vi "MultiScanDrift.vi"() -> ()   [LabVIEW 2014]
uses:
  <userlib>/Nanonis Prog Interface V5/Nanonis Prog Interface.lvlib
  shared/CorrelImages (SubVI)Single.vi
panel:
  in  "DC On":bool
  out "Y drift":i32
  out "X drift":i32
  in  "PLL switch delay":dbl=0.5 format="%_3p"
  out "DC active":bool
  in  "Drift correction Pixels":i32=256
  in  "Img Current":sgl=2.5e-11 format="%#_6p"
  in  "Img Bias (V)":sgl=0.02 format="%_2p"
  in  "Forward Speed":sgl=5e-10 format="%#_6p"
  in  "Backward Speed":sgl=8e-08 format="%#_6p"
  in  "Img Speed":sgl=3e-08 format="%#_6p"
  in  "Channel index (0-23)":u8(ring) items=["Current"=0, "Z (m)"=14]
  in  "Settling time (s)":dbl=0.7 format="%#_6p"
  in  "img bias":bool=TRUE
  in  "img bias":dbl=-0.0012 format="%#_6p"
  in  "img delay (s)":u32=1
  out "tipLift":dbl=1e-10 format="%#_6p"
  in  "TipLiftList":i32(listbox)
  in  "Const Height":bool=TRUE
  in  "CurrentList":i32(listbox)
  in  "BiasList":i32(listbox)
  out "Current":dbl=2.5e-11 format="%#_6p"
  out "Bias":dbl=0.02 format="%#_6p"
  # "Turn continuous scan off"
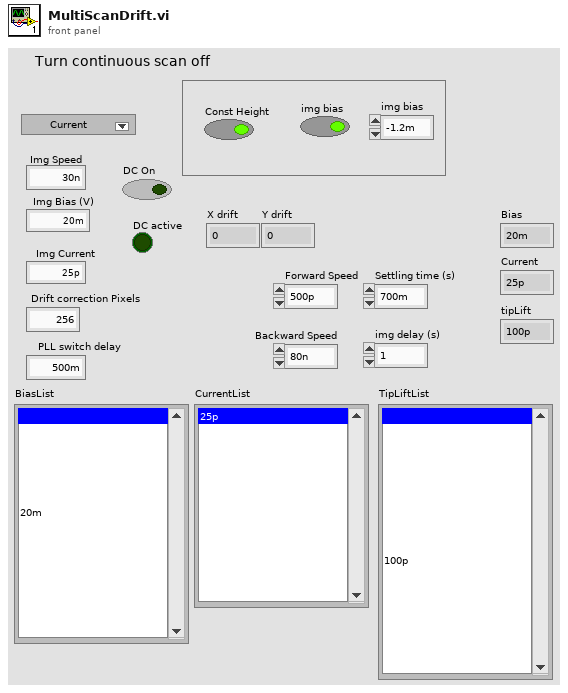
[diagram p1: front panel]
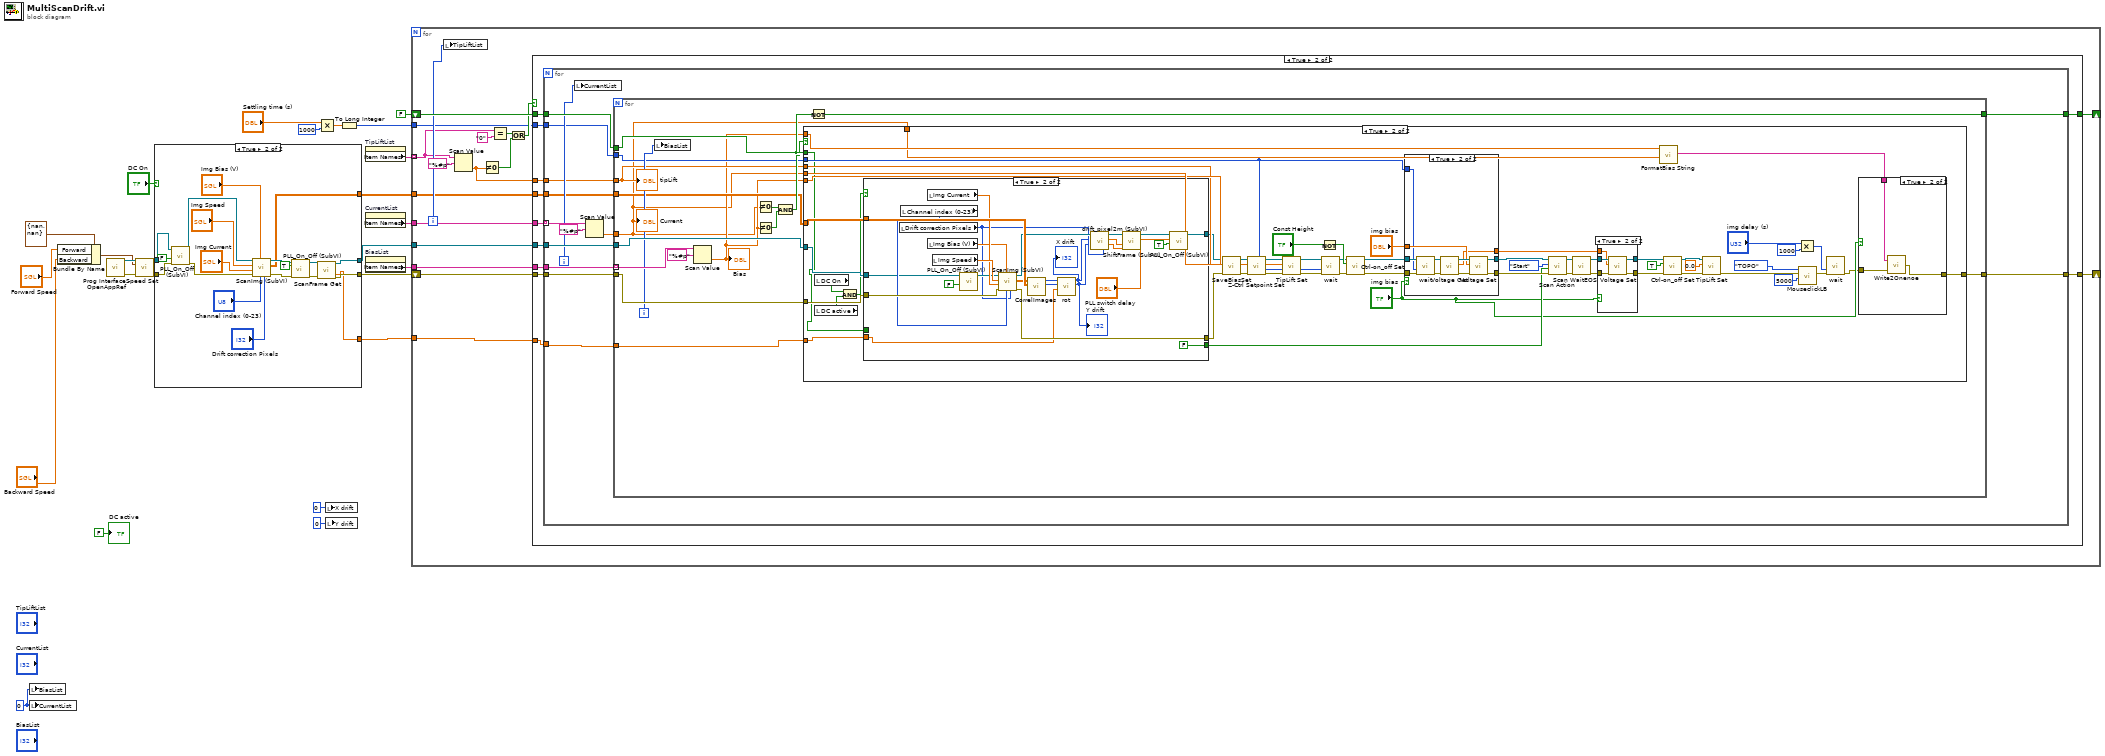
[diagram p0: block diagram]
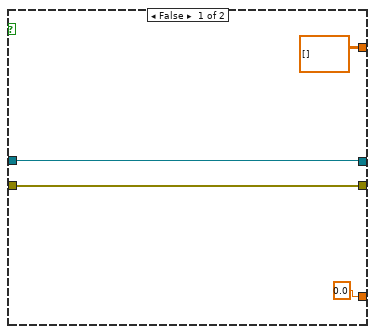
[diagram p2: hidden frame]
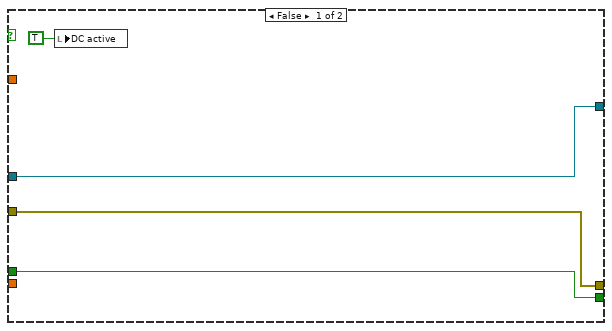
[diagram p6: hidden frame]
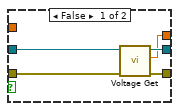
[diagram p8: hidden frame]
diagram:
  w25 = 0 ("BiasList")
  n1 = local write "BiasList"(w25) -> ()
  n2 = local write "CurrentList"(w25) -> ()
  n3 = Bundle By Name(cluster=cluster{"Forward":sgl, "Backward":sgl} {"Forward"=nan, "Backward"=nan} ("Speed (m/s)"), "Forward"="Forward Speed", "Backward"="Backward Speed") -> (w9:cluster{"Forward":sgl, "Backward":sgl})
  n4 = call <userlib>:"Prog Interface - OpenAppRef.vi"() -> ("Error out"=w10:errorcluster, "Application reference"=w11:refnum<vi>)  [unwired: 6 in]
  n5 = call <userlib>:"Speed Set.vi"("Application ref in"=w11, "Speed (m/s)"=w9, "error in (no error)"=w10) -> ("Application ref out"=w7:refnum<vi>, "error out"=w6:errorcluster)  [unwired: 11 in]
  n6 = case shown="True" "DC On" {
    tunnel: [w28 w32] -> w13
    tunnel: [w27 w31] -> w12
    tunnel: [dbl[][] [] ("Img") w41] -> w8
    tunnel: w7 -> [w28 w40]
    tunnel: w6 -> [w27 w38]
    tunnel: [sgl 0.0 ("Angle (deg)") w30] -> w1
    frame False {
    }
    frame True {
      n7 = call "PLL_On_Off (SubVI).vi"("error in (no error)"=w38, "Output ON/OFF (F=OFF)"=FALSE, "Application in"=w40) -> ("error out"=w37:errorcluster, "Application out"=w39:refnum<vi>)  [unwired: 7 in]
      n8 = call "ScanImg (SubVI).vi"("pixel"="Drift correction Pixels", "Channel index (0-23)"="Channel index (0-23)", "Bias (V)"="Img Bias (V)", "error in (no error)"=w37, "Current"="Img Current", "Img Speed"="Img Speed", "Application in"=w39) -> ("error out"=w44:errorcluster, "Img"=w41:dbl[][], "Application out"=w45:refnum<vi>)  [unwired: 2 in]
      n9 = call "PLL_On_Off (SubVI).vi"("error in (no error)"=w44, "Output ON/OFF (F=OFF)"=TRUE, "Application in"=w45) -> ("error out"=w33:errorcluster, "Application out"=w34:refnum<vi>)  [unwired: 7 in]
      n10 = call <userlib>:"ScanFrame Get.vi"("Application ref in"=w34, "error in (no error)"=w33) -> ("Application ref out"=w32:refnum<vi>, "Angle (deg)"=w30:sgl, "error out"=w31:errorcluster)  [unwired: 9 in, 2 out]
    }
  }
  n11 = Multiply(x="Settling time (s)", y=u32 1000) -> (x*y=w21:dbl)
  n12 = local write "X drift"(0 ("X drift")) -> ()
  n13 = local write "Y drift"(0 ("Y drift")) -> ()
  n14 = To Long Integer(number=w21) -> (32bit integer=w22:i32)
  n15 = property on="TipLiftList" class="LstBox (strict)"() -> ("Item Names"=w17:string[])  [unwired: 2 in, 2 out]
  n16 = property on="CurrentList" class="LstBox (strict)"() -> ("Item Names"=w18:string[])  [unwired: 2 in, 2 out]
  n17 = property on="BiasList" class="LstBox (strict)"() -> ("Item Names"=w19:string[])  [unwired: 2 in, 2 out]
  n18 = for {
    tunnel: w19 -> [w65]
    tunnel: w18 -> [w64]
    tunnel: w13 -> [w63]
    tunnel: w17 -> [w59] mode=indexing
    shift-right: [w53] -> _
    shift-left: FALSE ("Direction: up/down (T=up)") -> [w66]
    tunnel: w22 -> [w52]
    tunnel: w8 -> [w51]
    tunnel: w1 -> [w50]
    shift-right: [w49] -> _
    shift-left: w12 -> [w62]
    i -> [w60]
    n19 = local write "TipLiftList"(w60) -> ()
    n20 = Scan Value(string=w59, format string="%#p") -> (value=w58:dbl)  [unwired: 1 in, 1 out]
    n21 = Not Equal To 0?(x=w58) -> (x != 0?=w57:bool)
    n22 = Equal?(x=w59, y="0") -> (x = y?=w54:bool)
    n23 = Or(x=w54, y=w57) -> (x .or. y?=w56:bool)
    n24 = case shown="True" w56 {
      tunnel: w66 -> [w68 w79]
      tunnel: w65 -> [_ w78]
      tunnel: w64 -> [_ w77]
      tunnel: w63 -> [_ w76]
      tunnel: w62 -> [w67 w75]
      tunnel: w58 -> [_ w74]
      tunnel: [w68 w73] -> w53
      tunnel: w52 -> [_ w72]
      tunnel: w51 -> [_ w71]
      tunnel: w50 -> [_ w70]
      tunnel: [w67 w69] -> w49
      frame False {
      }
      frame True {
        n25 = for {
          tunnel: w79 -> [w93]
          tunnel: w76 -> [w92]
          tunnel: w75 -> [w91]
          tunnel: w78 -> [w90]
          tunnel: w77 -> [w88] mode=indexing
          tunnel: w74 -> [w85]
          tunnel: [w84] -> w73
          tunnel: w72 -> [w83]
          tunnel: w71 -> [w82]
          tunnel: w70 -> [w81]
          tunnel: [w80] -> w69
          i -> [w86]
          n26 = local write "CurrentList"(w86) -> ()
          n27 = Scan Value(string=w88, format string="%#p") -> (value=w87:dbl)  [unwired: 1 in, 1 out]
          n28 = for {
            tunnel: w90 -> [w105] mode=indexing
            tunnel: w92 -> [w107]
            tunnel: w91 -> [w106]
            tunnel: w87 -> [w95]
            tunnel: w85 -> [w100]
            tunnel: w93 -> [w109]
            tunnel: [w108] -> w84
            tunnel: w83 -> [w99]
            tunnel: w82 -> [w98]
            tunnel: w81 -> [w97]
            tunnel: [w94] -> w80
            i -> [w101]
            n29 = local write "BiasList"(w101) -> ()
            n30 = Scan Value(string=w105, format string="%#p") -> (value=w96:dbl)  [unwired: 1 in, 1 out]
            "Bias" <- w96
            n31 = Not Equal To 0?(x=w95) -> (x != 0?=w104:bool)
            n32 = Not Equal To 0?(x=w96) -> (x != 0?=w103:bool)
            n33 = Compound Arithmetic op=AND(w104, w103) -> (w102:bool)
            n34 = case shown="True" w102 {
              tunnel: w109 -> [_ w120]
              tunnel: w96 -> [_ w163]
              tunnel: w107 -> [_ w127]
              tunnel: w106 -> [w111 w126]
              tunnel: w95 -> [_ w166]
              tunnel: w100 -> [_ w153]
              tunnel: w99 -> [_ w129]
              tunnel: w98 -> [_ w128]
              tunnel: w97 -> [_ w118]
              tunnel: w96 -> [_ w117]
              tunnel: w95 -> [_ w116]
              tunnel: [w111 w112] -> w94
              frame False {
              }
              frame True {
                n35 = local read "DC On"() -> (w122:bool)
                n36 = local read "DC active"() -> (w123:bool)
                n37 = And(x=w122, y=w123) -> (x .and. y?=w121:bool)
                n38 = case shown="True" w121 {
                  tunnel: w128 -> [_ w200]
                  tunnel: w127 -> [w173 w188]
                  tunnel: w126 -> [w174 w199]
                  tunnel: [w174 w198] -> w125
                  tunnel: [w173 w185] -> w124
                  tunnel: [w171 FALSE ("Direction: up/down (T=up)")] -> w119
                  tunnel: w120 -> [w171 _]
                  tunnel: w118 -> [_ w179]
                  frame False {
                    n39 = local write "DC active"(TRUE ("DC active")) -> ()
                  }
                  frame True {
                    n40 = local read "Drift correction Pixels"() -> (w182:i32)
                    n41 = local read "Channel index (0-23)"() -> (w193:u8)
                    n42 = local read "Img Current"() -> (w195:sgl)
                    n43 = local read "Img Bias (V)"() -> (w194:sgl)
                    n44 = local read "Img Speed"() -> (w196:sgl)
                    n45 = call "PLL_On_Off (SubVI).vi"("Output ON/OFF (F=OFF)"=FALSE, "Application in"=w188) -> ("Application out"=w187:refnum<vi>)  [unwired: 8 in, 1 out]
                    n46 = call "ScanImg (SubVI).vi"("pixel"=w182, "Channel index (0-23)"=w193, "Bias (V)"=w194, "error in (no error)"=w199, "Current"=w195, "Img Speed"=w196, "Application in"=w187) -> ("error out"=w198:errorcluster, "Img"=w197:dbl[][], "Application out"=w189:refnum<vi>)  [unwired: 2 in]
                    n47 = call-poly "CorrelImages.vi"("Ref Array"=w200, "New Image"=w197) -> ("Y drift"=w176:i32, "X drift"=w178:i32)  [unwired: 6 in, 2 out]
                    n48 = call "rot.vi"("angle"=w179, "y"=w176, "x"=w178) -> ("y'"=w175:i32, "x'"=w177:i32)  [unwired: 7 in]
                    "X drift" <- w177
                    "Y drift" <- w175
                    n49 = call "drift_pixel2m (SubVI).vi"("Application in"=w189, "X drift"=w177, "Y drift"=w175, "Drift correction Pixels"=w182) -> ("Application out"=w190:refnum<vi>, "x drift"=w192:sgl, "y drift"=w191:sgl)  [unwired: 2 in, 1 out]
                    n50 = call "ShiftFrame (SubVI).vi"("Y shift"=w191, "X shift"=w192, "Application in"=w190) -> ("Application out"=w186:refnum<vi>)  [unwired: 8 in]
                    n51 = call "PLL_On_Off (SubVI).vi"("Output ON/OFF (F=OFF)"=TRUE, 10:"PLL switch delay", "Application in"=w186) -> ("Application out"=w185:refnum<vi>)  [unwired: 7 in, 1 out]
                  }
                }
                n52 = call "SaveBiasSet.vi"("Application ref in"=w124, "Bias (V)"=w163, "error in (no error)"=w125) -> ("Application ref out"=w165:refnum<vi>, "Error out"=w164:errorcluster)  [unwired: 6 in]
                n53 = call <userlib>:"Z-Ctrl Setpoint Set.vi"("error in (no error)"=w164, "Z Controller setpoint"=w166, "Application ref in"=w165) -> ("error out"=w154:errorcluster, "Application ref out"=w156:refnum<vi>)  [unwired: 7 in]
                n54 = call <userlib>:"TipLift Set.vi"("error in (no error)"=w154, "TipLift (m)"=w153, "Application ref in"=w156) -> ("error out"=w130:errorcluster, "Application ref out"=w155:refnum<vi>)  [unwired: 7 in]
                n55 = Not(x="Const Height") -> (.not. x?=w159:bool)
                n56 = call "wait.vi"("error in"=w130, "milliseconds to wait"=w129, "application reference in"=w155) -> ("error out"=w131:errorcluster, "application reference out"=w132:refnum<vi>)  [unwired: 7 in]
                n57 = call <userlib>:"Ctrl-on_off Set.vi"("error in (no error)"=w131, "Z Controller ON/OFF"=w159, "Application ref in"=w132) -> ("error out"=w148:errorcluster, "Application ref out"=w150:refnum<vi>)  [unwired: 7 in]
                n58 = case shown="True" "img bias" {
                  tunnel: w150 -> [w212 w214]
                  tunnel: [w211 w221] -> w149
                  tunnel: w148 -> [w208 w217]
                  tunnel: [w209 w220] -> w147
                  tunnel: "img bias" -> [_ w219]
                  tunnel: [w210 w218] -> w145
                  tunnel: w129 -> [_ w213]
                  frame False {
                    n59 = call <userlib>:"Voltage Get.vi"("error in (no error)"=w208, "Application ref in"=w212) -> ("error out"=w209:errorcluster, "Bias (V)"=w210:sgl, "Application ref out"=w211:refnum<vi>)  [unwired: 7 in]
                  }
                  frame True {
                    n60 = call "wait.vi"("error in"=w217, "milliseconds to wait"=w213, "application reference in"=w214) -> ("error out"=w216:errorcluster, "application reference out"=w215:refnum<vi>)  [unwired: 7 in]
                    n61 = call <userlib>:"Voltage Get.vi"("error in (no error)"=w216, "Application ref in"=w215) -> ("error out"=w223:errorcluster, "Bias (V)"=w218:sgl, "Application ref out"=w222:refnum<vi>)  [unwired: 7 in]
                    n62 = call <userlib>:"Voltage Set.vi"("Error in (no error)"=w223, "Bias (V)"=w219, "Application ref in"=w222) -> ("Error out"=w220:errorcluster, "Application ref out"=w221:refnum<vi>)  [unwired: 7 in]
                  }
                }
                n63 = call <userlib>:"Scan Action.vi"("error in (no error)"=w147, "Direction: up/down (T=up)"=w119, "Scan action (Start)"=enum16{"Start", "Stop", "Pause", "Resume"}."Start", "Application ref in"=w149) -> ("error out"=w162:errorcluster, "Application ref out"=w161:refnum<vi>)  [unwired: 5 in]
                n64 = call <userlib>:"Scan WaitEOS.vi"("error in (no error)"=w162, "Application ref in"=w161) -> ("error out"=w143:errorcluster, "Application ref out"=w144:refnum<vi>)  [unwired: 5 in, 2 out]
                n65 = case shown="True" "img bias" {
                  tunnel: w144 -> [w202 w205]
                  tunnel: [w202 w207] -> w142
                  tunnel: [w201 w206] -> w141
                  tunnel: w143 -> [w201 w204]
                  tunnel: w145 -> [_ w203]
                  frame False {
                  }
                  frame True {
                    n66 = call <userlib>:"Voltage Set.vi"("Error in (no error)"=w204, "Bias (V)"=w203, "Application ref in"=w205) -> ("Error out"=w206:errorcluster, "Application ref out"=w207:refnum<vi>)  [unwired: 7 in]
                  }
                }
                n67 = call "FormatBias String.vi"("current"=w116, "bias"=w117) -> ("resulting string"=w113:string)  [unwired: 9 in]
                n68 = call <userlib>:"Ctrl-on_off Set.vi"("error in (no error)"=w141, "Z Controller ON/OFF"=TRUE, "Application ref in"=w142) -> ("error out"=w140:errorcluster, "Application ref out"=w139:refnum<vi>)  [unwired: 7 in]
                n69 = call <userlib>:"TipLift Set.vi"("error in (no error)"=w140, "TipLift (m)"=sgl 0.0, "Application ref in"=w139) -> ("error out"=w152:errorcluster)  [unwired: 7 in, 1 out]
                n70 = Multiply(x="img delay (s)", y=u32 1000) -> (x*y=w134:u32)
                n71 = call "MouseclickLB.vi"("nMilliseconds"=5000, "error in (no error)"=w152, "Click"=enum16{"Header", "TOPO", "STS", "GRID"}."TOPO") -> ("error out"=w133:errorcluster)  [unwired: 8 in]
                n72 = call "wait.vi"("error in"=w133, "milliseconds to wait"=w134) -> ("error out"=w114:errorcluster)  [unwired: 8 in, 1 out]
                n73 = case shown="True" "img bias" {
                  tunnel: w114 -> [w167 w170]
                  tunnel: w113 -> [_ w169]
                  tunnel: [w167 w168] -> w112
                  frame False {
                  }
                  frame True {
                    n74 = call "Write2Onenoe.vi"("error in (no error)"=w170, "strSendText"=w169) -> ("error out"=w168:errorcluster)
                  }
                }
              }
            }
            n75 = Not(x=w109) -> (.not. x?=w108:bool)
            "Current" <- w95
            "tipLift" <- w100
          }
        }
      }
    }
  }
  "DC active" <- FALSE ("DC active")
